vi "Sgl_GetProperty.vi"(5 "Error In":errorcluster) -> (15 "Property":dbl, 19 "Error Out":errorcluster)   [LabVIEW 2020]
uses:
  <resource>/Framework/Providers/Open_GDS/ClassProviders/Provider_EndevoGOOP300/Templates/SingletonTemplate/SingletonTemplate.lvclass
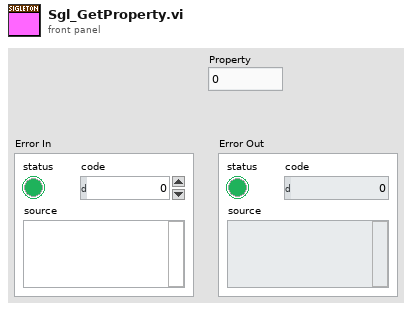
[diagram p1: front panel]
types:
  T1 = typedef "SingletonTemplate.lvclass/ObjectAttributes.ctl" = cluster{"Attribute1":dbl}
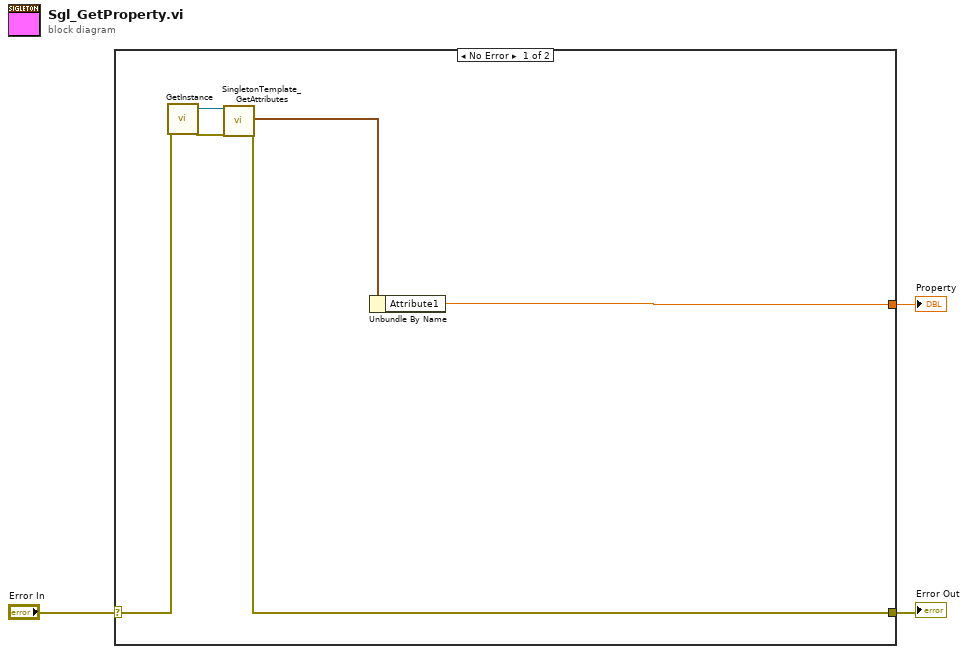
[diagram p0: block diagram]
diagram:
  n1 = case shown="No Error" "Error In" {
    selector: "Error In" -> [w4 w10]
    tunnel: [w8 w10] -> w2
    tunnel: [w7 _] -> w1
    frame No Error {
      n2 = call <resource>:"GetInstance.vi"("error in (no error)"=w4) -> ("reference out"=w6:refnum<class "SingletonTemplate.lvclass">, "error out"=w5:errorcluster)  [unwired: 17 in]
      n3 = call <resource>:"SingletonTemplate_GetAttributes.vi"("reference in"=w6, "error in (no error)"=w5) -> ("Attributes"=w9:T1, "error out"=w8:errorcluster)  [unwired: 14 in, 2 out]
      n4 = Unbundle By Name(w9) -> ("Attribute1"=w7:dbl)
    }
    frame Error {
    }
  }
  "Error Out" <- w2
  "Property" <- w1
